vi "Actor Last Ack.vi"(10 "Nested Actor":refnum<class "Actor.lvclass">, 11 "Self Actor in":refnum<class "Self Actor.lvclass">) -> (3 "Self Actor out":refnum<class "Self Actor.lvclass">)   [LabVIEW 2021, in "jettl.lvlib" / "Self Actor.lvclass"]
uses:
  Self Actor.lvclass
  Actor/Actor.lvclass
  Self Actor.lvclass/Self Actor.ctl
  jettl.lvlib
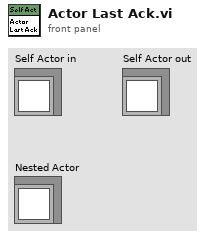
[diagram p1: front panel]
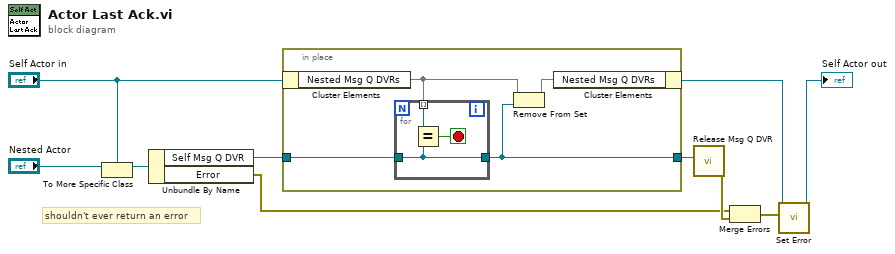
[diagram p0: block diagram]
diagram:
  # "shouldn't ever return an error"
  n1 = To More Specific Class(target class="Self Actor in", reference="Nested Actor") -> (specific class reference=w10:refnum<class "Self Actor.lvclass">)  [unwired: 1 in, 1 out]
  n2 = Unbundle By Name(w10) -> ("Self Msg Q DVR"=w8:refnum<data-value>, "Error"=w5:errorcluster)
  n3 = in-place {
    in-place-border: w8 -> [w12]
    in-place-border: [w11] -> w7
    n4 = in-place-cluster #1("Self Actor in") -> ("Nested Msg Q DVRs"=w14:set{refnum<data-value>})
    n5 = for {
      tunnel: w12 -> [w15]
      tunnel: w14 -> [w16] mode=indexing
      tunnel: [w15] -> w11
      stop <- w17 stop-if-true
      n6 = Equal?(x=w16, y=w15) -> (x = y?=w17:bool)
    }
    n7 = Remove From Set(10:w11, 11:w14) -> (3:w13:set{refnum<data-value>})  [unwired: 1 out]
    n8 = in-place-cluster #1("Nested Msg Q DVRs"=w13) -> (w4:refnum<class "Self Actor.lvclass">)
  }
  n9 = call "Release Msg Q DVR.vi"("Msg Q DVR"=w7) -> ("error out"=w6:errorcluster)  [unwired: 10 in]
  n10 = Merge Errors(w5, w6) -> (w2:errorcluster)
  n11 = call-dynamic "Set Error.vi"("Error"=w2, "Self Actor in"=w4) -> ("Self Actor out"=→"Self Actor out":refnum<class "Self Actor.lvclass">)  [unwired: 9 in]
